vi "Log20mA.vi"(8 "error in (no error)":errorcluster, 11 "LotData in":refnum<class "LotData.lvclass">) -> (0 "error out":errorcluster, 1 "area":i32, 2 "reverse":dbl, 3 "LotData out":refnum<class "LotData.lvclass">)   [LabVIEW 2012, in "LotData.lvclass"]
uses:
  LotData.lvclass
  <vilib>/addons/database/NI_Database_API.lvlib
  <vilib>/addons/database/Connection.llb/DB Tools Open Connec (Path).vi
  <vilib>/addons/database/Auxilliary.llb/DB Tools Parameter Dir.ctl
  <vilib>/addons/database/Auxilliary.llb/DB Tools DataTypes.ctl
  <vilib>/addons/database/Auxilliary.llb/DB Tools Parameter Info.ctl
  <vilib>/addons/database/Command.llb/Cmd Set Parameter Value (C).vi
  <vilib>/addons/database/Command.llb/Cmd Execute.vi
  <vilib>/addons/database/Recordset.llb/Rec Destroy - Command.vi
  <vilib>/addons/database/Command.llb/Cmd Delete.vi
panel:
  out "Area":i32
  out "knee":dbl
  out "s? t:f":dbl
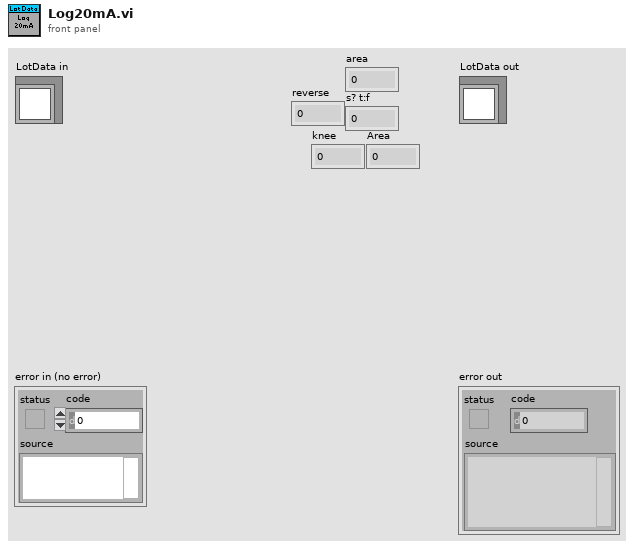
[diagram p1: front panel]
types:
  T1 = typedef "NI_Database_API.lvlib/DB Tools Parameter Info.ctl" = cluster{"parameter name":string, "type":T2, "direction":T3, "value":variant}
  T2 = typedef "NI_Database_API.lvlib/DB Tools DataTypes.ctl" = enum16{"String", "Long (I32)", "Single (SGL)", "Double (DBL)", "Date/Time", "Binary"}
  T3 = typedef "NI_Database_API.lvlib/DB Tools Parameter Dir.ctl" = enum32{"Input", "Output", "Input/Output", "Return Value"}
  T4 = typedef "LotData.lvclass/LotData_Current.ctl" = cluster{"area":i32, "Data":cluster{"wl":dbl, "power":dbl, "voltage":dbl, "knee":dbl, "reverse":dbl}}
  T5 = typedef "MeasurementType.ctl" = enum16{"Initial", "Final"}
  T6 = typedef "NI_Database_API.lvlib/Conn ObjectReference.ctl" = refnum<k1>
  T7 = typedef "NI_Database_API.lvlib/Cmd ObjectReference.ctl" = refnum<k1>
  T8 = cluster{"wl":dbl, "power":dbl, "voltage":dbl, "knee":dbl, "reverse":dbl}
  T9 = typedef "NI_Database_API.lvlib/Cmd-Rec Object Reference.ctl" = refnum<k1>
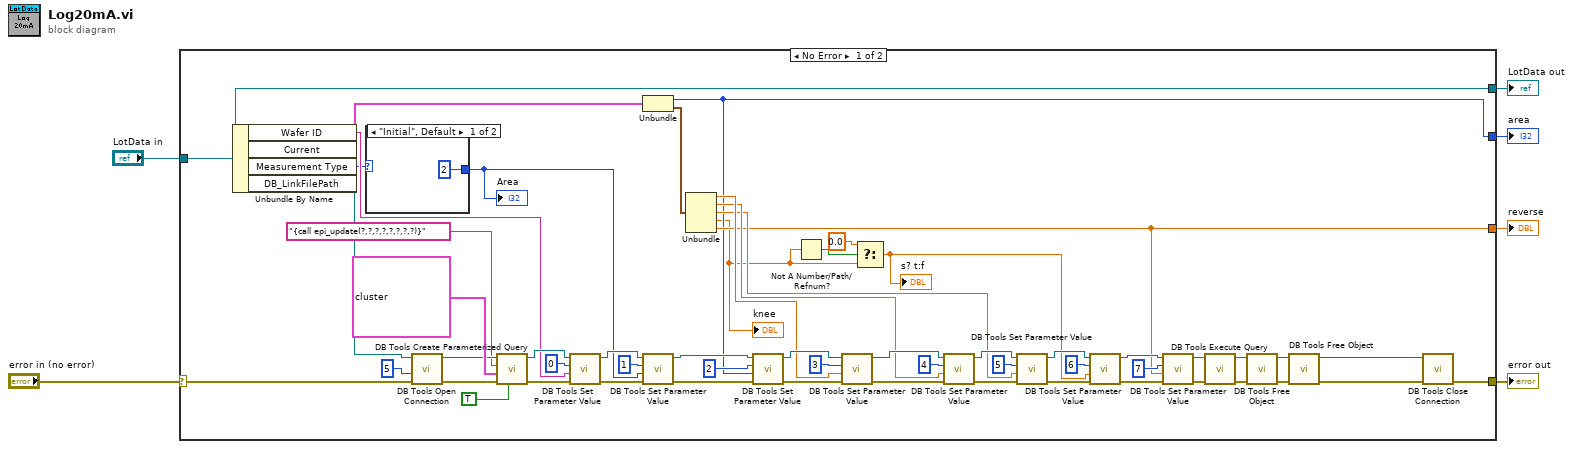
[diagram p0: block diagram]
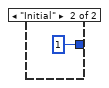
[diagram p2: hidden frame]
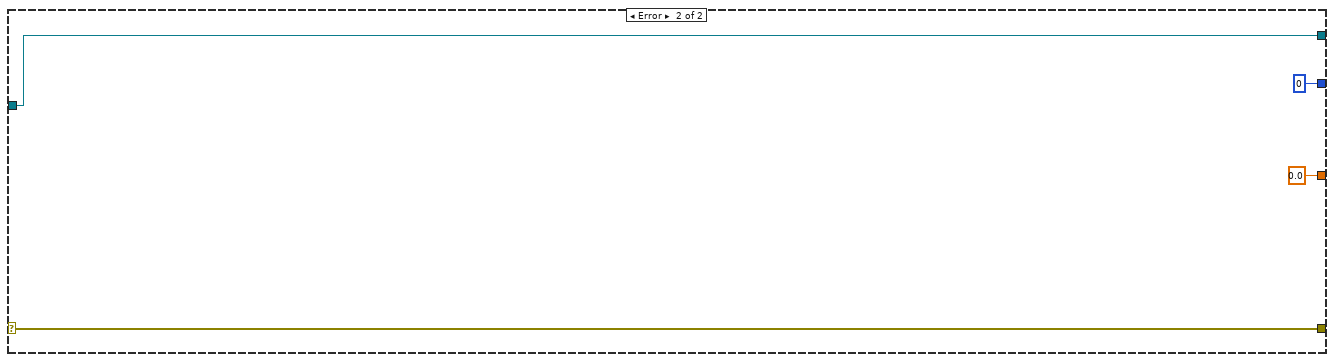
[diagram p3: hidden frame]
diagram:
  n1 = case shown="No Error" "error in (no error)" {
    selector: "error in (no error)" -> [w25 w68]
    tunnel: [w16 w68] -> w5
    tunnel: [w13 w67] -> w3
    tunnel: "LotData in" -> [w13 w67]
    tunnel: [w15 0.0 ("reverse")] -> w2
    tunnel: [w14 0 ("area")] -> w1
    frame No Error {
      n2 = Unbundle By Name(w13) -> ("Wafer ID"=w22:string, "Current"=w24:T4, "Measurement Type"=w21:T5, "DB_LinkFilePath"=w8:path)
      n3 = case shown="Default, \"After\"" w21 {
        tunnel: [2 1] -> w20
        frame "Initial", Default {
        }
        frame "Initial" {
        }
      }
      "Area" <- w20
      n4 = call-poly <vilib>:"DB Tools Open Connection.vi"("error in (no error)"=w25, "connection timeout (15)"=5, "connection information"=w8) -> ("error out"=w59:errorcluster, "connection reference"=w60:T6)  [unwired: 5 in]
      n5 = call <vilib>:"DB Tools Create Parameterized Query.vi"("stored procedure? (F)"=TRUE, "error in (no error)"=w59, "parameters"=T1[] [{"parameter name"="wafer", "type"=enum."String", "direction"=enum."Input", "value"=variant}, {"parameter name"="test", "type"=enum."Single (SGL)", "direction"=enum."Input", "value"=variant}, {"parameter name"="area", "type"=enum."Single (SGL)", "direction"=enum."Input", "value"=variant}, {"parameter name"="wl", "type"=enum."Double (DBL)", "direction"=enum."Input", "value"=variant}, {"parameter name"="power", "type"=enum."Double (DBL)", "direction"=enum."Input", "value"=variant}, {"parameter name"="voltage", "type"=enum."Double (DBL)", "direction"=enum."Input", "value"=variant}, {"parameter name"="knee", "type"=enum."Double (DBL)", "direction"=enum."Input", "value"=variant}, {"parameter name"="reverse", "type"=enum."Double (DBL)", "direction"=enum."Input", "value"=variant}], "SQL query"="{call epi_update(?,?,?,?,?,?,?,?)}", "connection reference"=w60) -> ("error out"=w56:errorcluster, "command reference"=w55:T7)  [unwired: 2 in, 1 out]
      n6 = call-poly <vilib>:"DB Tools Set Parameter Value.vi"("error in (no error)"=w56, "value"=w22, "parameter index"=0, "command reference"=w55) -> ("error out"=w26:errorcluster, "command reference out"=w41:T7)  [unwired: 4 in]
      n7 = Unbundle(w24) -> ("area"=w14:i32, "Data"=w23:T8)
      n8 = call-poly <vilib>:"DB Tools Set Parameter Value.vi"("error in (no error)"=w26, "value"=w20, "parameter index"=1, "command reference"=w41) -> ("error out"=w27:errorcluster, "command reference out"=w40:T7)  [unwired: 4 in]
      n9 = Unbundle(w23) -> ("wl"=w19:dbl, "power"=w18:dbl, "voltage"=w17:dbl, "knee"=w10:dbl, "reverse"=w15:dbl)
      "knee" <- w10
      n10 = call-poly <vilib>:"DB Tools Set Parameter Value.vi"("error in (no error)"=w27, "value"=w14, "parameter index"=2, "command reference"=w40) -> ("error out"=w28:errorcluster, "command reference out"=w39:T7)  [unwired: 4 in]
      n11 = Not A Number/Path/Refnum?(number/path/refnum=w10) -> (NaN/Path/Refnum?=w12:bool)
      n12 = call-poly <vilib>:"DB Tools Set Parameter Value.vi"("error in (no error)"=w28, "value"=w19, "parameter index"=3, "command reference"=w39) -> ("error out"=w29:errorcluster, "command reference out"=w38:T7)  [unwired: 4 in]
      n13 = Select(t=0.0, s=w12, f=w10) -> (s? t:f=w9:dbl)
      "s? t:f" <- w9
      n14 = call-poly <vilib>:"DB Tools Set Parameter Value.vi"("error in (no error)"=w29, "value"=w18, "parameter index"=4, "command reference"=w38) -> ("error out"=w30:errorcluster, "command reference out"=w37:T7)  [unwired: 4 in]
      n15 = call-poly <vilib>:"DB Tools Set Parameter Value.vi"("error in (no error)"=w30, "value"=w17, "parameter index"=5, "command reference"=w37) -> ("error out"=w31:errorcluster, "command reference out"=w36:T7)  [unwired: 4 in]
      n16 = call-poly <vilib>:"DB Tools Set Parameter Value.vi"("error in (no error)"=w31, "value"=w9, "parameter index"=6, "command reference"=w36) -> ("error out"=w32:errorcluster, "command reference out"=w35:T7)  [unwired: 4 in]
      n17 = call-poly <vilib>:"DB Tools Set Parameter Value.vi"("error in (no error)"=w32, "value"=w15, "parameter index"=7, "command reference"=w35) -> ("error out"=w33:errorcluster, "command reference out"=w34:T7)  [unwired: 4 in]
      n18 = call-poly <vilib>:"DB Tools Execute Query.vi"("error in (no error)"=w33, "command reference"=w34) -> ("error out"=w52:errorcluster, "command-recordset reference"=w53:T9)  [unwired: 6 in]
      n19 = call-poly <vilib>:"DB Tools Free Object.vi"("error in (no error)"=w52, "command-recordset reference"=w53) -> ("error out"=w54:errorcluster, "command reference"=w51:T7)  [unwired: 8 in]
      n20 = call-poly <vilib>:"DB Tools Free Object.vi"("error in (no error)"=w54, "command reference"=w51) -> ("error out"=w49:errorcluster, "connection reference"=w50:T6)  [unwired: 8 in]
      n21 = call <vilib>:"DB Tools Close Connection.vi"("error in (no error)"=w49, "connection reference"=w50) -> ("error out"=w16:errorcluster)  [unwired: 5 in]
    }
    frame Error {
    }
  }
  "error out" <- w5
  "LotData out" <- w3
  "reverse" <- w2
  "area" <- w1
